vi "Example Zoom.vi"() -> ()   [LabVIEW 2020, in "LcPictureBox.lvclass"]
uses:
  LcPictureBox.lvclass
  System.Windows.Forms
  <vilib>/Utility/miscctls.llb/LVPoint32TypeDef.ctl
  Pen.ctl
  SmoothingMode.ctl
panel:
  in  "PictureBox":refnum<k24>(container)
  out "WheelPosition":cluster{"X":i32, "Y":i32}
  out "MouseDown":cluster{"X":i32, "Y":i32}
  in  "Origin":cluster{"x":sgl, "y":sgl}
  in  "ZoomAtMouse":bool
  out "MousePosition(raw)":cluster{"X":i32, "Y":i32}
  in  "ScaleToFit":bool
  in  "ScaleFactor(1)":dbl=1.0 min=-5.0 max=5.0 step=0.1 format="%#.1f"
  in  "Stop":bool
  out "Updating":u32
  out "Drawing":u32
  out "error out":errorcluster
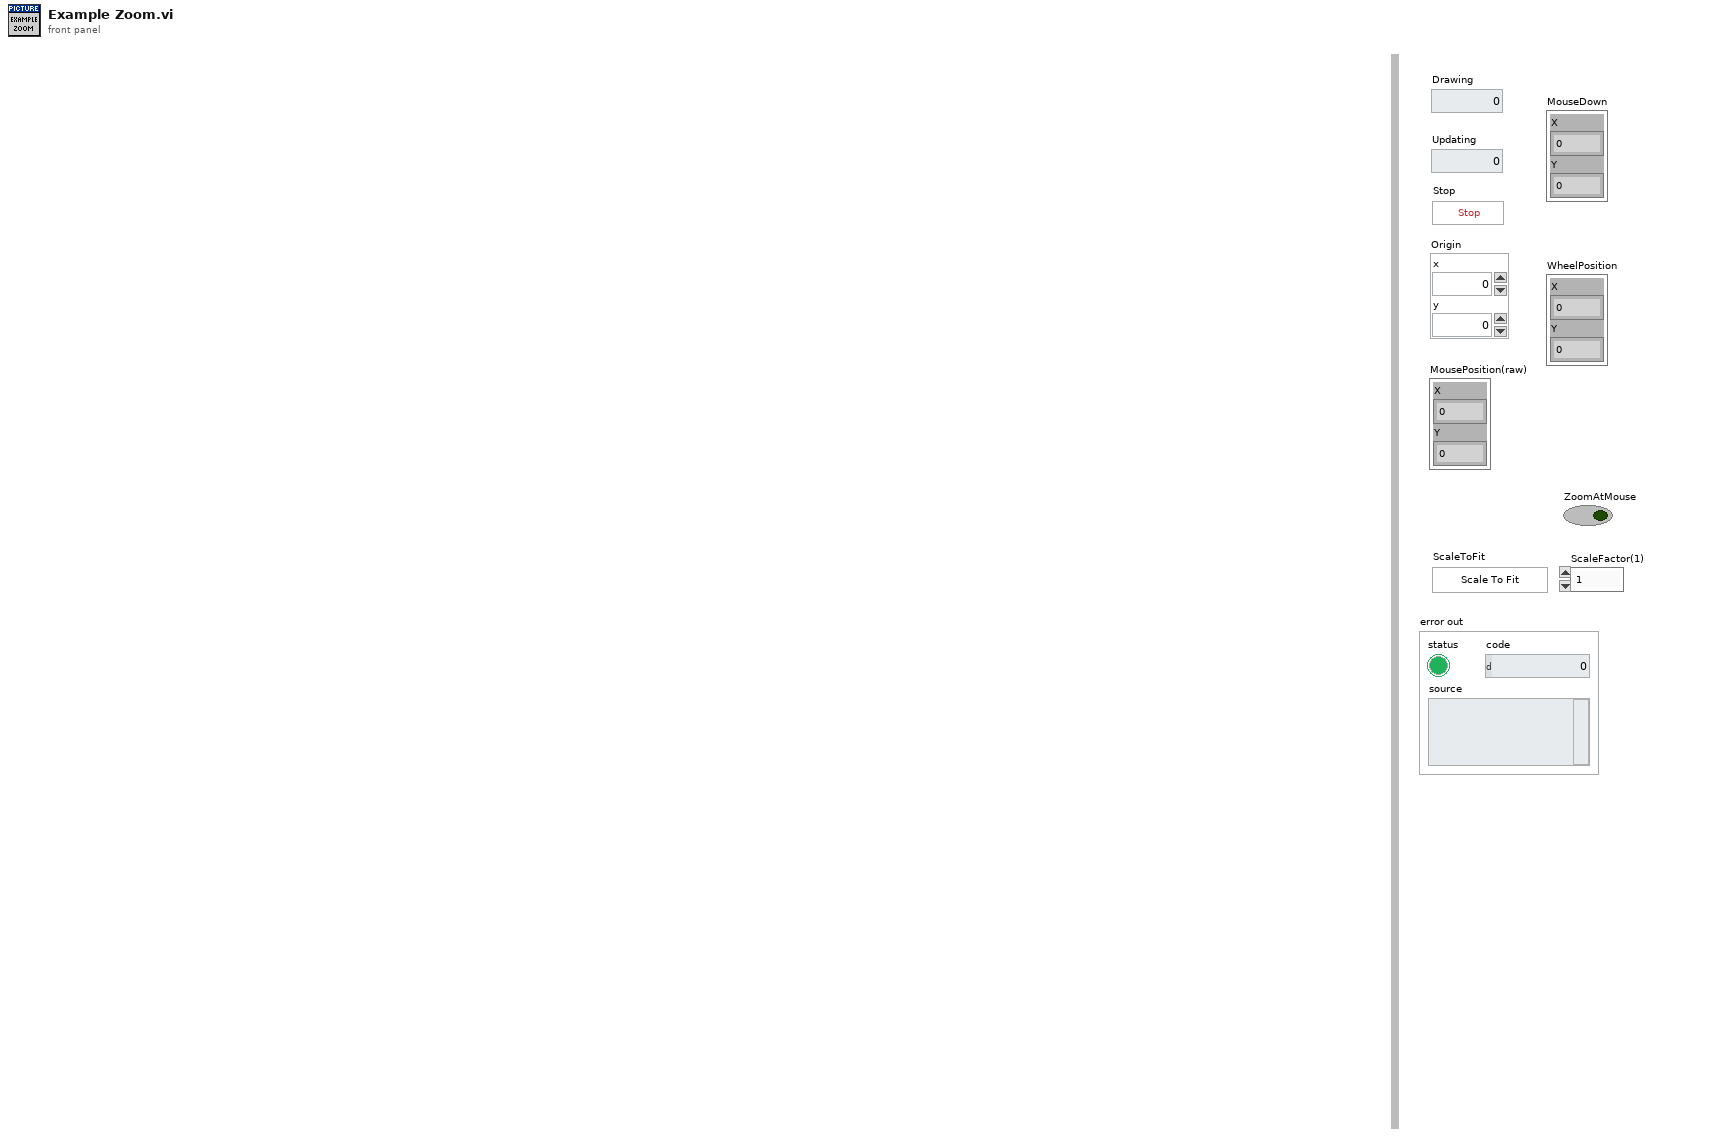
[diagram p1: front panel]
types:
  T1 = typedef "LVPoint32TypeDef.ctl" = cluster{"Horizontal":i32, "Vertical":i32}
  T2 = cluster{"Coords":T1, "MouseDown":bool, "PlatMods":cluster{"Shift":bool, "Ctrl":bool, "Alt":bool, "Cmd":bool, "Opt":bool}}
  T3 = typedef "LcPictureBox.lvclass/Pen.ctl" = cluster{"Width":u16, "Style":enum32{"Solid", "Dash", "Dot", "DashDot", "DashDotDot"}}
  T4 = typedef "LcPictureBox.lvclass/SmoothingMode.ctl" = enum16{"None", "HighSpeed", "HighQuality", "AntiAlias"}
  T5 = cluster{"Shift":bool, "Ctrl":bool, "Alt":bool, "Cmd":bool, "Opt":bool}
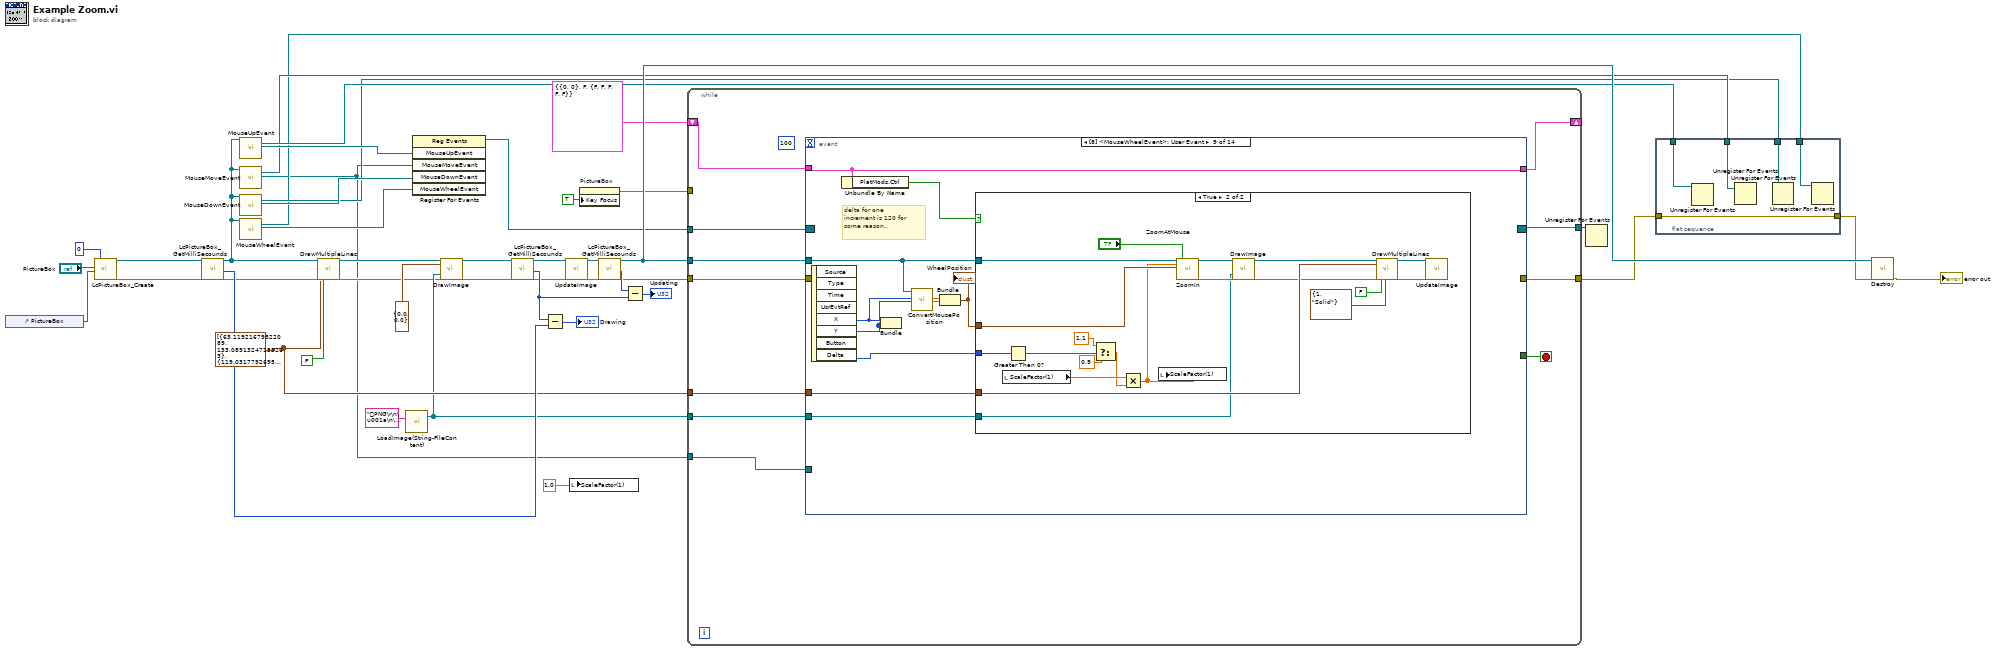
[diagram p0: block diagram]
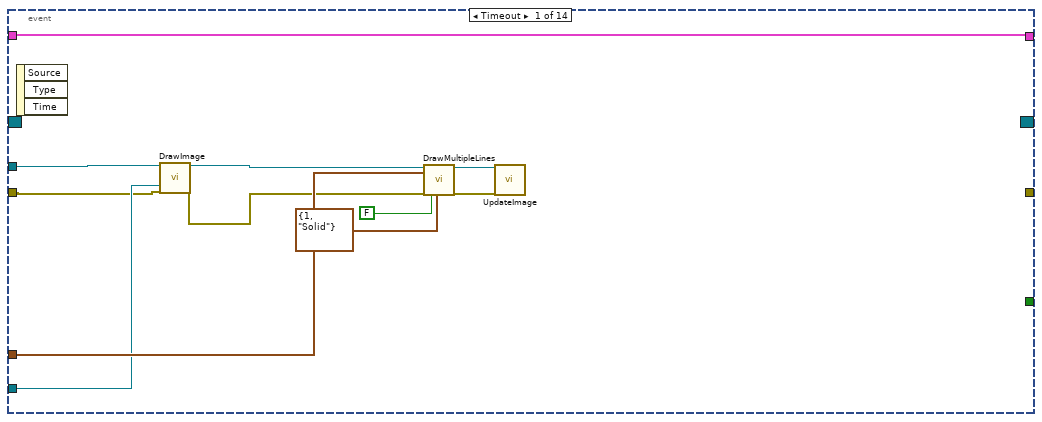
[diagram p2: hidden frame]
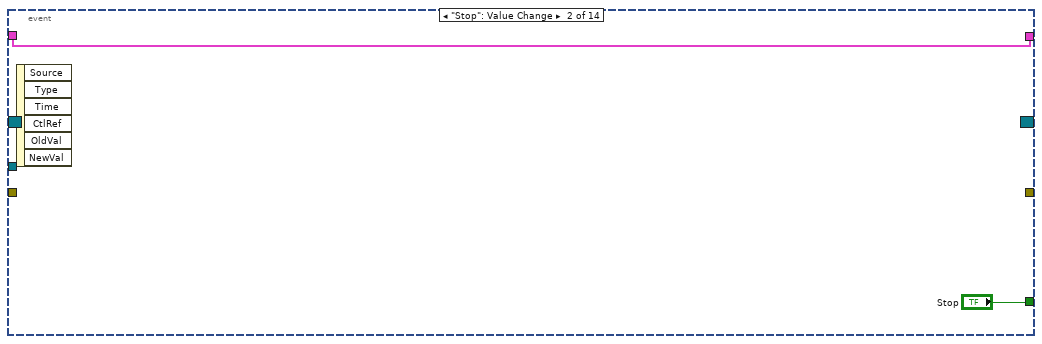
[diagram p3: hidden frame]
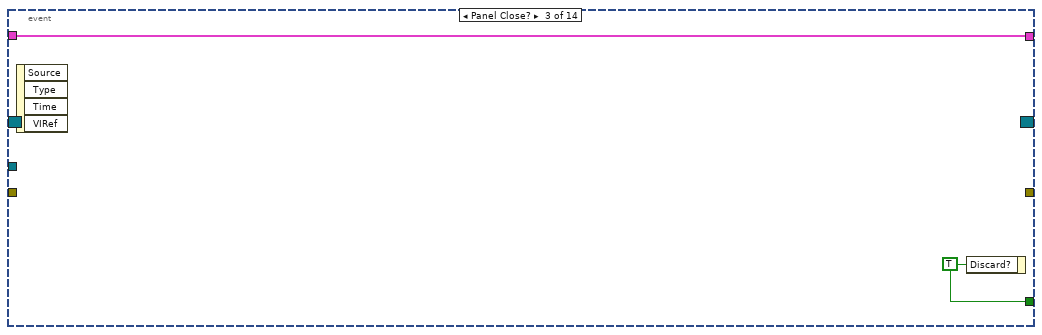
[diagram p4: hidden frame]
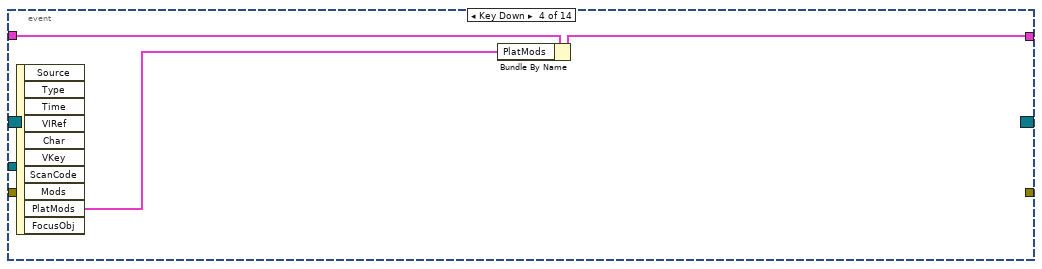
[diagram p5: hidden frame]
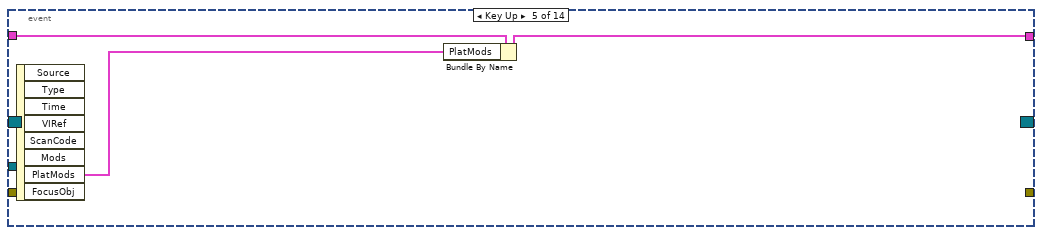
[diagram p6: hidden frame]
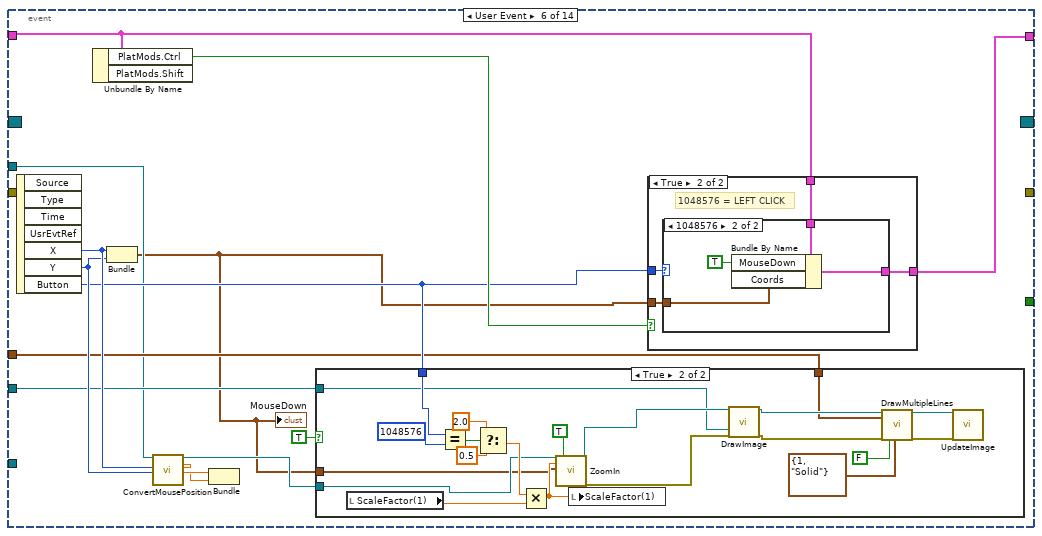
[diagram p7: hidden frame]
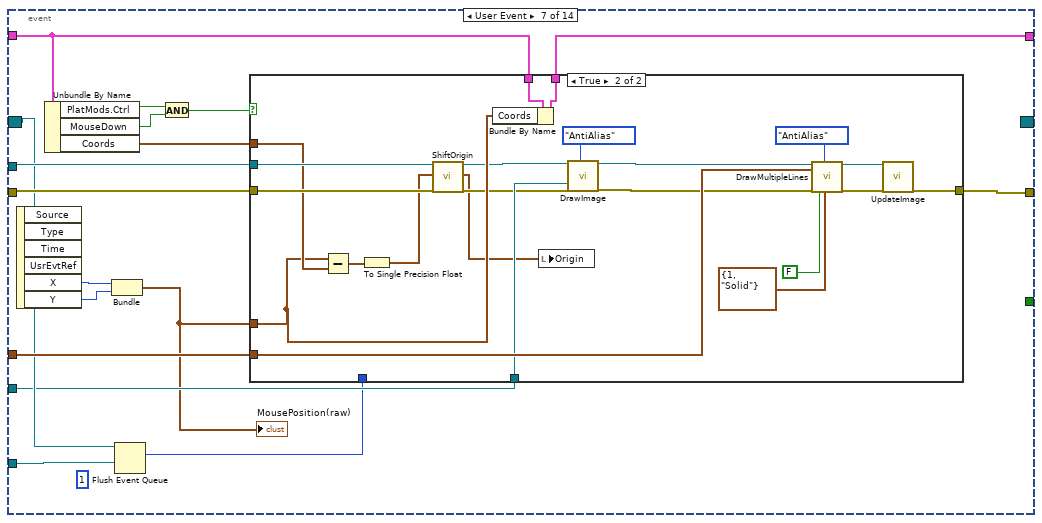
[diagram p11: hidden frame]
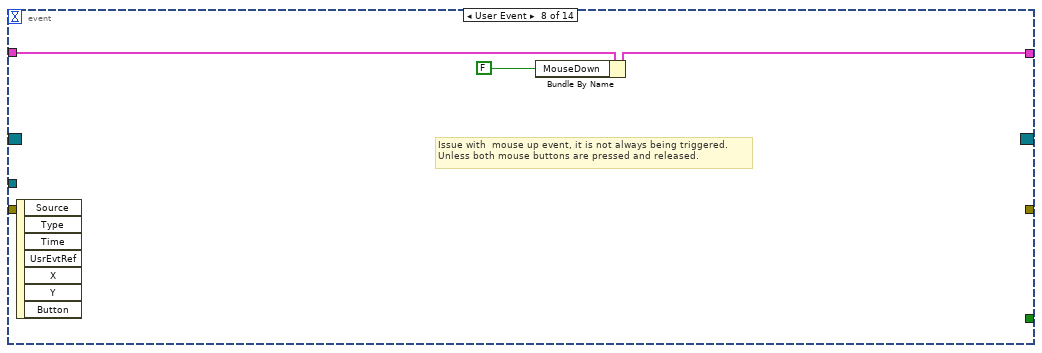
[diagram p13: hidden frame]
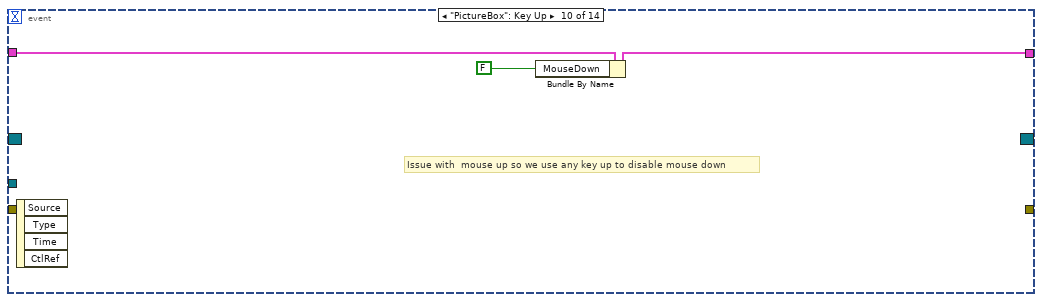
[diagram p15: hidden frame]
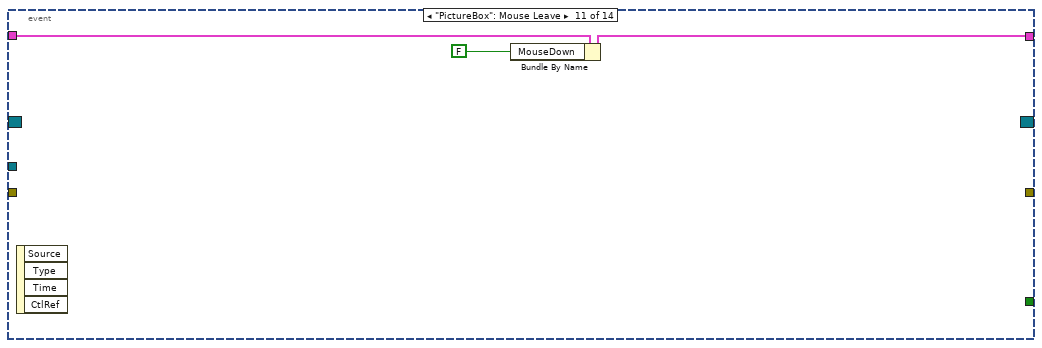
[diagram p16: hidden frame]
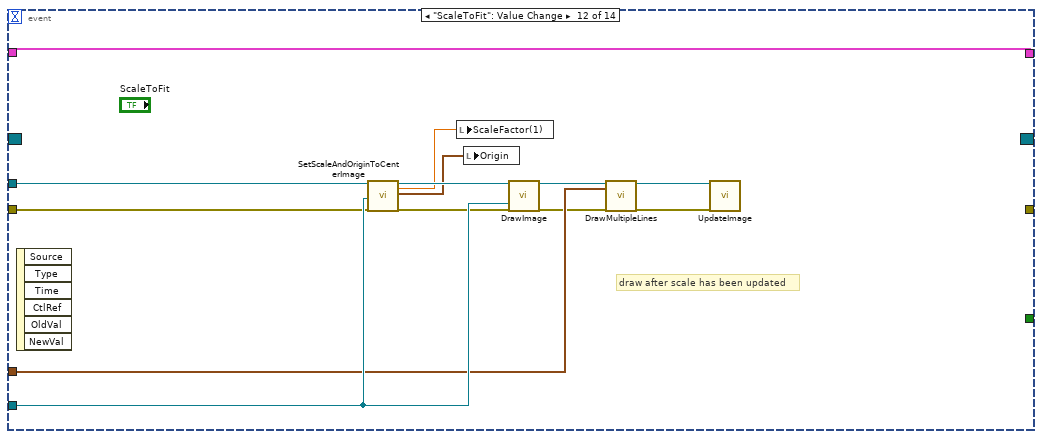
[diagram p17: hidden frame]
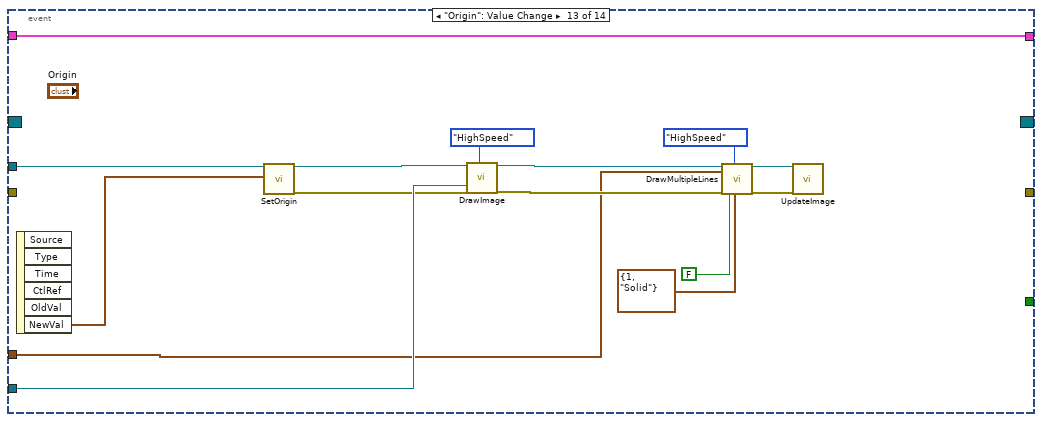
[diagram p18: hidden frame]
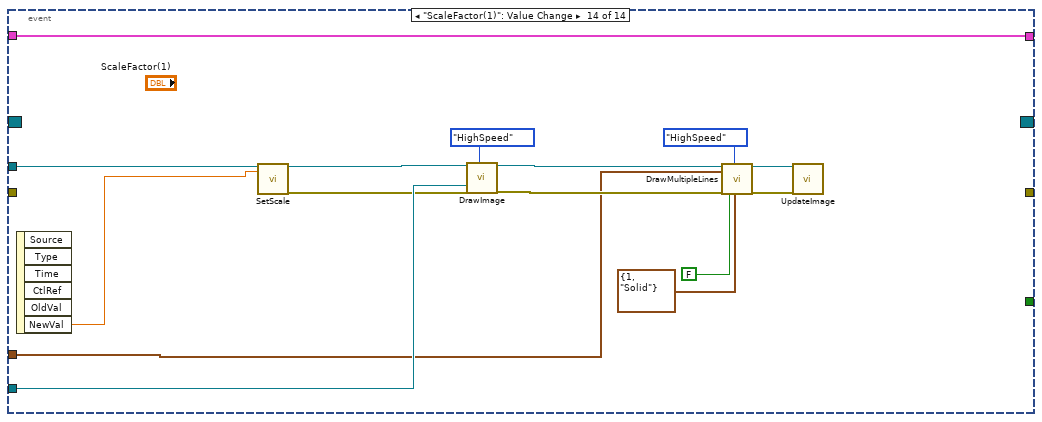
[diagram p19: hidden frame]
diagram:
  w25 = cluster{dbl, dbl}[] [{63.11921679522089, 133.08913247155263}, {119.03177926954152, 161.04541370871294}, {174.94434174386214, 133.08913247155263}, {202.90062298102245, 189.00169494587325}, {174.94434174386214, 244.91425742019388}, {119.03177926954152, 216.95797618303357}, {63.11921679522089, 244.91425742019388}, {35.16293555806058, 189.00169494587325}, {63.11921679522089, 133.08913247155263}]
  n1 = control-ref of="PictureBox"() -> (w39:refnum<vi>)
  n2 = call "LcPictureBox_Create.vi"("PictureBox"="PictureBox", "PictureBoxActiveXReference"=w39, "CacheNumberOfPensAndColors(0)"=0 ("CacheNumberOfPensAndColors(1000)")) -> ("reference out"=w3:refnum<class "LcPictureBox.lvclass">, "Error Out"=w1:errorcluster)  [unwired: 14 in, 1 out]
  n3 = call "LcPictureBox_GetMilliSecounds.vi"("error in (no error)"=w1) -> ("msValue"=w38:u32, "error out"=w31:errorcluster)  [unwired: 17 in]
  n4 = call-dynamic "MouseUpEvent.vi"("reference in"=w3) -> ("Event Callback Refnum"=w15:refnum<k27>, "MouseUpEvent"=w19:refnum<user-event>)  [unwired: 15 in, 2 out]
  n5 = call-dynamic "MouseMoveEvent.vi"("reference in"=w3) -> ("Event Callback Refnum"=w14:refnum<k27>, "MouseMoveEvent"=w4:refnum<user-event>)  [unwired: 15 in, 2 out]
  n6 = call-dynamic "MouseDownEvent.vi"("reference in"=w3) -> ("Event Callback Refnum"=w13:refnum<k27>, "MouseDownEvent"=w18:refnum<user-event>)  [unwired: 15 in, 2 out]
  n7 = call-dynamic "MouseWheelEvent.vi"("reference in"=w3) -> ("Event Callback Refnum"=w9:refnum<k27>, "MouseWheelEvent"=w8:refnum<user-event>)  [unwired: 15 in, 2 out]
  n8 = call-dynamic "DrawMultipleLines.vi"("reference in"=w3, "LineEndPoints"=w25, "Error In"=w31, "Fill(False)"=FALSE ("x > y?")) -> ("reference out"=w28:refnum<class "LcPictureBox.lvclass">, "Error Out"=w6:errorcluster)  [unwired: 14 in]
  n9 = call "LoadImage(String-FileContent).vi"("ImageFileContent"="PNG\r\n\u001a\n\u0000\u0000\u0000\rIHDR\u0000\u0000\u0000ß\u0000\u0000\u0000â\b\u0003\u0000\u0000\u0000ùÃâm\u0000\u0000\u0000PLTEÿÚ\u001cÿÿÿ\u0000\u0000\u0000ÿ×\u0000ÿýôÿÙ\u0000ÿá\u001dÿÝ\u001cÿß\u001d¡\u0012n\u000eUI\tÉ¬\u0016îÌ\u001aÿã\u001dÿÚ\u0015:1\u0006¼ \u0015ÿùãÿäoÿìÿï²ÿý÷ÿÞBÿûîÿ÷Ûÿð¸ÿôÉÿöÔÿåzÿêÿéÿæÿá_ÿßKÿí©ÿòÀÿÞGÿàTÿÜ2ÿêÿäsÿùáöÓ\u001b\u0011we\rÿÝ8ÿâfl\\\f'!\u0004J?\btÙ\u0000\u0000\u0006\u0001IDATxíÝSÓL\u0010\u0007ð«á@}(\u0014ÆÒP\u0014\u0015Ô÷ÿâ\\[´K²¹ìÞþ\u0018¿ÿ1Óéä3´ý6Éºí¸Ý\u001föªéòqu}~~}u²¼<æ:&Ììø¦w÷¾ÜÆûâä#ßqaå¯ªi®²øª^øä\u0015.\u0012_,÷X\u000fot¶¾(ÏpësÏ_»ÂÅ\u0019ï1ÉÆ÷Å·òÐ_2\u001fez6¾NÞZøù8S³öMû|A8å>Ô¤¬}\u001dï¾]ágîMHðUý¿¾°Ô'\f¾9Ð\u0017§Ü\u0007<0Á\u0007æÕÿÒx7ã>äA©}\u0017\u0003|AxwÃ}Ð\u0003â@zµï\nòéùLøPq\u001f80nÐÛoGx®Cè&{mÿZ÷\bëOÜ\u0007\u000fH²/\bW\u0017Üß\u0011¾ ¼ºç\u0006ôd/\b\u001fe×4#}Ax\"Y8Ú'¼¦Að\u0011.Uâ\u0013\\Ó ùÄÖ4h¾0\u0000\u000b\u0014\"úD\u0016Q¨>5\r²O\u0010Ý'¬\"ðªiH|µÐ\t\u0011\u0012ùÄ\u0014QT>)5\rOFMCéPÓÐúðµ¦¡öq\u0017Qô>Þ\"*...") -> ("ImageOut"=w7:refnum<k24>)  [unwired: 16 in, 2 out]
  n10 = register-events(w19, w4, w18, w8) -> (reference out=w17:refnum<event-registration>)  [unwired: 2 in, 1 out]
  n11 = call-dynamic "DrawImage.vi"("reference in"=w28, "UpperLeftCorner(0,0)"=cluster{"x":sgl, "y":sgl} {"x"=0.0, "y"=0.0} ("UpperLeftCorner"), "Image"=w7, "Error In"=w6) -> ("reference out"=w27:refnum<class "LcPictureBox.lvclass">, "Error Out"=w5:errorcluster)  [unwired: 14 in]
  n12 = call "LcPictureBox_GetMilliSecounds.vi"("error in (no error)"=w5) -> ("msValue"=w37:u32, "error out"=w33:errorcluster)  [unwired: 17 in]
  n13 = Subtract(x=w37, y=w38) -> (x-y=→"Drawing":u32)
  n14 = call-dynamic "UpdateImage.vi"("reference in"=w27, "Error In"=w33) -> ("reference out"=w24:refnum<class "LcPictureBox.lvclass">, "Error Out"=w34:errorcluster)  [unwired: 14 in, 2 out]
  n15 = local write "ScaleFactor(1)"(1.0 ("ScaleFactor(1)")) -> ()
  n16 = property on="PictureBox" class="AXCont"("Key Focus"=TRUE) -> (error out=w20:errorcluster)  [unwired: 2 in, 1 out]
  n17 = call "LcPictureBox_GetMilliSecounds.vi"("error in (no error)"=w34) -> ("msValue"=w36:u32, "error out"=w23:errorcluster)  [unwired: 17 in]
  n18 = Subtract(x=w36, y=w37) -> (x-y=→"Updating":u32)
  n19 = while {
    tunnel: w24 -> [w51]
    tunnel: w25 -> [w50]
    tunnel: w7 -> [w49]
    tunnel: w23 -> [w48]
    tunnel: [w47] -> w11
    shift-right: [w46] -> _
    shift-left: T2 {"Coords"={"Horizontal"=0, "Vertical"=0}, "MouseDown"=FALSE, "PlatMods"={"Shift"=FALSE, "Ctrl"=FALSE, "Alt"=FALSE, "Cmd"=FALSE, "Opt"=FALSE}} -> [w44]
    tunnel: w20 -> [_]
    tunnel: w17 -> [w43]
    tunnel: [w45] -> w16
    tunnel: w4 -> [w42]
    stop <- w52 stop-if-true
    (unwired) 100
    n20 = event shown="[8] <MouseWheelEvent>: User Event" {
      selector: w43 -> [_ _ _ _ _ _ w122 _ _ _ _ _ _ _]
      dyn-events: [_ _ _ _ _ _ _ _ _ _ _ _ _ _] -> w45
      timeout: _ -> [_ _ _ _ _ _ _ _ _ _ _ _ _ _]
      tunnel: [_ "Stop" w66 _ _ _ _ _ _ _ _ _ _ _] -> w52
      tunnel: w51 -> [w57 _ _ _ _ w79 w135 _ w167 _ _ w206 w215 w231]
      tunnel: w50 -> [w61 _ _ _ _ w80 w128 _ w173 _ _ w203 w217 w232]
      tunnel: w49 -> [w56 _ _ _ _ w81 w121 _ w170 _ _ w209 w218 w233]
      tunnel: w48 -> [w55 _ _ _ _ _ w134 _ _ _ _ w207 _ _]
      tunnel: [_ _ _ _ _ _ w133 _ _ _ _ _ _ _] -> w47
      tunnel: [w58 w64 w67 w69 w72 w87 w130 w161 w172 w195 w198 w212 w227 w242] -> w46
      tunnel: w44 -> [w58 w64 w67 w70 w73 w86 w127 w162 w172 w196 w199 w212 w227 w242]
      tunnel: w42 -> [_ _ _ _ _ _ w123 _ _ _ _ _ _ _]
      event Timeout {
        n21 = event-data() -> ()  [unwired: 1 in, 3 out]
        n22 = call-dynamic "DrawImage.vi"("reference in"=w57, "Image"=w56, "Error In"=w55) -> ("reference out"=w53:refnum<class "LcPictureBox.lvclass">, "Error Out"=w54:errorcluster)  [unwired: 15 in]
        n23 = call-dynamic "DrawMultipleLines.vi"("reference in"=w53, "LineEndPoints"=w61, "Error In"=w54, "Fill(False)"=FALSE ("x > y?"), "Pen(Width=1, Solid)"=T3 {"Width"=1, "Style"=enum."Solid"}) -> ("reference out"=w60:refnum<class "LcPictureBox.lvclass">, "Error Out"=w59:errorcluster)  [unwired: 13 in]
        n24 = call-dynamic "UpdateImage.vi"("reference in"=w60, "Error In"=w59) -> ()  [unwired: 14 in, 4 out]
      }
      event "Stop": Value Change {
        n25 = event-data() -> ()  [unwired: 1 in, 6 out]
      }
      event Panel Close? {
        w66 = TRUE ("Discard?")
        n26 = event-data() -> ()  [unwired: 1 in, 4 out]
        n27 = event-data("Discard?"=w66) -> ()  [unwired: 1 in, 1 out]
      }
      event Key Down {
        n28 = event-data() -> ("PlatMods"=w68:T5)  [unwired: 1 in, 9 out]
        n29 = Bundle By Name(cluster=w70, "PlatMods"=w68) -> (w69:T2)
      }
      event Key Up {
        n30 = event-data() -> ("PlatMods"=w71:T5)  [unwired: 1 in, 7 out]
        n31 = Bundle By Name(cluster=w73, "PlatMods"=w71) -> (w72:T2)
      }
      event User Event {
        n32 = event-data() -> ("X"=w84:i32, "Y"=w83:i32, "Button"=w82:i32)  [unwired: 1 in, 4 out]
        n33 = Unbundle By Name(w86) -> ("PlatMods.Ctrl"=w85:bool)  [unwired: 1 out]
        n34 = Bundle("X"=w84, "Y"=w83) -> (w74:cluster{"X":i32, "Y":i32})  [unwired: 1 in]
        "MouseDown" <- w74
        n35 = call-dynamic "ConvertMousePosition.vi"("reference in"=w79, "X"=w84, "Y"=w83) -> ("reference out"=w78:refnum<class "LcPictureBox.lvclass">, "X-Out"=w77:sgl, "Y-Out"=w76:sgl)  [unwired: 13 in, 1 out]
        n36 = Bundle("X-Out"=w77, "Y-Out"=w76) -> ()  [unwired: 1 in, 1 out]
        n37 = case shown="True" TRUE {
          tunnel: w82 -> [_ w104]
          tunnel: w81 -> [_ w91]
          tunnel: w80 -> [_ w90]
          tunnel: w78 -> [_ w89]
          tunnel: w74 -> [_ w88]
          frame False {
          }
          frame True {
            n38 = local read "ScaleFactor(1)"() -> (w100:dbl)
            n39 = Equal?(x=w104, y=1048576) -> (x = y?=w107:bool)
            n40 = Select(t=2.0, s=w107, f=0.5) -> (s? t:f=w102:dbl)
            n41 = Multiply(x=w102, y=w100) -> (x*y=w101:dbl)
            n42 = call-dynamic "ZoomIn.vi"("reference in"=w89, "NewScaleValue"=w101, "MousePosition(scaled)"=w88, "ZoomAtMouse"=TRUE) -> ("reference out"=w93:refnum<class "LcPictureBox.lvclass">, "Error Out"=w92:errorcluster)  [unwired: 12 in, 2 out]
            n43 = local write "ScaleFactor(1)"(w101) -> ()
            n44 = call-dynamic "DrawImage.vi"("reference in"=w93, "Image"=w91, "Error In"=w92) -> ("reference out"=w94:refnum<class "LcPictureBox.lvclass">, "Error Out"=w95:errorcluster)  [unwired: 15 in]
            n45 = call-dynamic "DrawMultipleLines.vi"("reference in"=w94, "LineEndPoints"=w90, "Error In"=w95, "Fill(False)"=FALSE ("x > y?"), "Pen(Width=1, Solid)"=T3 {"Width"=1, "Style"=enum."Solid"}) -> ("reference out"=w97:refnum<class "LcPictureBox.lvclass">, "Error Out"=w96:errorcluster)  [unwired: 13 in]
            n46 = call-dynamic "UpdateImage.vi"("reference in"=w97, "Error In"=w96) -> ()  [unwired: 14 in, 4 out]
          }
        }
        n47 = case shown="True" w85 {
          tunnel: w86 -> [w109 w113]
          tunnel: [w109 w112] -> w87
          tunnel: w82 -> [_ w111]
          tunnel: w74 -> [_ w110]
          frame False {
          }
          frame True {
            # "1048576 = LEFT CLICK"
            n48 = case shown="1048576" w111 {
              tunnel: w113 -> [w114 w118]
              tunnel: [w114 w117] -> w112
              tunnel: w110 -> [_ w115]
              frame 0, Default {
              }
              frame 1048576 {
                n49 = Bundle By Name(cluster=w118, "MouseDown"=TRUE, "Coords"=w115) -> (w117:T2)
              }
            }
          }
        }
      }
      event User Event {
        (unwired) 1 ("keep most recent")
        n50 = event-data() -> ("X"=w131:i32, "Y"=w132:i32)  [unwired: 1 in, 4 out]
        n51 = Unbundle By Name(w127) -> ("PlatMods.Ctrl"=w126:bool, "MouseDown"=w125:bool, "Coords"=w129:T1)
        n52 = Bundle("X"=w131, "Y"=w132) -> (w119:cluster{"X":i32, "Y":i32})  [unwired: 1 in]
        "MousePosition(raw)" <- w119
        n53 = Flush Event Queue(0:w122, 2:w123) -> (9:w120:u32)  [unwired: 4 in, 2 out]
        n54 = And(x=w126, y=w125) -> (x .and. y?=w124:bool)
        n55 = case shown="True" w124 {
          tunnel: w135 -> [_ w159]
          tunnel: w134 -> [w137 w158]
          tunnel: [w137 w146] -> w133
          tunnel: [w136 w156] -> w130
          tunnel: w127 -> [w136 w157]
          tunnel: w119 -> [_ w154]
          tunnel: w129 -> [_ w155]
          tunnel: w128 -> [_ w147]
          tunnel: w121 -> [_ w143]
          tunnel: w120 -> [_ _]
          frame False {
          }
          frame True {
            n56 = Subtract(x=w154, y=w155) -> (x-y=w153:T1)
            n57 = To Single Precision Float(number=w153) -> (single precision float=w152:cluster{"Horizontal":sgl, "Vertical":sgl})
            n58 = call-dynamic "ShiftOrigin.vi"("reference in"=w159, "Delta(raw)"=w152, "Error In"=w158) -> ("reference out"=w144:refnum<class "LcPictureBox.lvclass">, "Origin"=w138:cluster{"x":sgl, "y":sgl}, "Error Out"=w142:errorcluster)  [unwired: 14 in]
            n59 = Bundle By Name(cluster=w157, "Coords"=w154) -> (w156:T2)
            n60 = local write "Origin"(w138) -> ()
            n61 = call-dynamic "DrawImage.vi"("reference in"=w144, "Image"=w143, "Error In"=w142, "SmoothingMode(AntiAlias)"=SmoothingMode."AntiAlias" ("SmoothingMode")) -> ("reference out"=w141:refnum<class "LcPictureBox.lvclass">, "Error Out"=w140:errorcluster)  [unwired: 14 in]
            n62 = call-dynamic "DrawMultipleLines.vi"("reference in"=w141, "LineEndPoints"=w147, "Error In"=w140, "Fill(False)"=FALSE ("x > y?"), "SmoothingMode(AntiAlias)"=SmoothingMode."AntiAlias", "Pen(Width=1, Solid)"=T3 {"Width"=1, "Style"=enum."Solid"}) -> ("reference out"=w149:refnum<class "LcPictureBox.lvclass">, "Error Out"=w148:errorcluster)  [unwired: 12 in]
            n63 = call-dynamic "UpdateImage.vi"("reference in"=w149, "Error In"=w148) -> ("Error Out"=w146:errorcluster)  [unwired: 14 in, 3 out]
          }
        }
      }
      event User Event {
        # "Issue with  mouse up event, it is not always being triggered.\nUnless both mouse buttons are pressed and released."
        n64 = event-data() -> ()  [unwired: 1 in, 7 out]
        n65 = Bundle By Name(cluster=w162, "MouseDown"=FALSE) -> (w161:T2)
      }
      event User Event {
        # "delta for one increment is 120 for some reason.."
        n66 = event-data() -> ("X"=w169:i32, "Y"=w168:i32, "Delta"=w163:i32)  [unwired: 1 in, 5 out]
        n67 = Unbundle By Name(w172) -> ("PlatMods.Ctrl"=w171:bool)
        n68 = Bundle("X"=w169, "Y"=w168) -> ()  [unwired: 1 in, 1 out]
        n69 = call-dynamic "ConvertMousePosition.vi"("reference in"=w167, "X"=w169, "Y"=w168) -> ("X-Out"=w166:sgl, "Y-Out"=w164:sgl)  [unwired: 13 in, 2 out]
        n70 = Bundle("X-Out"=w166, "Y-Out"=w164) -> (w165:cluster{"X-Out":sgl, "Y-Out":sgl})  [unwired: 1 in]
        "WheelPosition" <- w165
        n71 = case shown="True" w171 {
          tunnel: w167 -> [_ w188]
          tunnel: w173 -> [_ w189]
          tunnel: w165 -> [_ w187]
          tunnel: w170 -> [_ w184]
          tunnel: w163 -> [_ w178]
          frame False {
          }
          frame True {
            n72 = local read "ScaleFactor(1)"() -> (w176:dbl)
            n73 = Greater Than 0?(x=w178) -> (x > 0?=w177:bool)
            n74 = Select(t=1.1, s=w177, f=0.9) -> (s? t:f=w175:dbl)
            n75 = Multiply(x=w176, y=w175) -> (x*y=w174:dbl)
            n76 = local write "ScaleFactor(1)"(w174) -> ()
            n77 = call-dynamic "ZoomIn.vi"("reference in"=w188, "NewScaleValue"=w174, "MousePosition(scaled)"=w187, "ZoomAtMouse"="ZoomAtMouse") -> ("reference out"=w186:refnum<class "LcPictureBox.lvclass">, "Error Out"=w185:errorcluster)  [unwired: 12 in, 2 out]
            n78 = call-dynamic "DrawImage.vi"("reference in"=w186, "Image"=w184, "Error In"=w185) -> ("reference out"=w182:refnum<class "LcPictureBox.lvclass">, "Error Out"=w183:errorcluster)  [unwired: 15 in]
            n79 = call-dynamic "DrawMultipleLines.vi"("reference in"=w182, "LineEndPoints"=w189, "Error In"=w183, "Fill(False)"=FALSE ("x > y?"), "Pen(Width=1, Solid)"=T3 {"Width"=1, "Style"=enum."Solid"}) -> ("reference out"=w191:refnum<class "LcPictureBox.lvclass">, "Error Out"=w190:errorcluster)  [unwired: 13 in]
            n80 = call-dynamic "UpdateImage.vi"("reference in"=w191, "Error In"=w190) -> ()  [unwired: 14 in, 4 out]
          }
        }
      }
      event "PictureBox": Key Up {
        # "Issue with  mouse up so we use any key up to disable mouse down"
        n81 = event-data() -> ()  [unwired: 1 in, 4 out]
        n82 = Bundle By Name(cluster=w196, "MouseDown"=FALSE) -> (w195:T2)
      }
      event "PictureBox": Mouse Leave {
        n83 = event-data() -> ()  [unwired: 1 in, 4 out]
        n84 = Bundle By Name(cluster=w199, "MouseDown"=FALSE) -> (w198:T2)
      }
      event "ScaleToFit": Value Change {
        # "draw after scale has been updated"
        n85 = event-data() -> ()  [unwired: 1 in, 6 out]
        n86 = call-dynamic "SetScaleAndOriginToCenterImage.vi"("reference in"=w206, "Image"=w209, "Error In"=w207) -> ("reference out"=w211:refnum<class "LcPictureBox.lvclass">, "ScaleFactorUsed"=w210:sgl, "OriginUsed"=w200:cluster{"x":sgl, "y":sgl}, "Error Out"=w208:errorcluster)  [unwired: 13 in]
        n87 = local write "ScaleFactor(1)"(w210) -> ()
        n88 = local write "Origin"(w200) -> ()
        n89 = call-dynamic "DrawImage.vi"("reference in"=w211, "Image"=w209, "Error In"=w208) -> ("reference out"=w205:refnum<class "LcPictureBox.lvclass">, "Error Out"=w202:errorcluster)  [unwired: 15 in]
        n90 = call-dynamic "DrawMultipleLines.vi"("reference in"=w205, "LineEndPoints"=w203, "Error In"=w202) -> ("reference out"=w204:refnum<class "LcPictureBox.lvclass">, "Error Out"=w201:errorcluster)  [unwired: 15 in]
        n91 = call-dynamic "UpdateImage.vi"("reference in"=w204, "Error In"=w201) -> ()  [unwired: 14 in, 4 out]
      }
      event "Origin": Value Change {
        n92 = event-data() -> ("NewVal"=w216:cluster{"x":sgl, "y":sgl})  [unwired: 1 in, 5 out]
        n93 = call-dynamic "SetOrigin.vi"("reference in"=w215, "Origin"=w216) -> ("reference out"=w214:refnum<class "LcPictureBox.lvclass">, "Error Out"=w213:errorcluster)  [unwired: 16 in]
        n94 = call-dynamic "DrawImage.vi"("reference in"=w214, "Image"=w218, "Error In"=w213, "SmoothingMode(AntiAlias)"=SmoothingMode."HighSpeed" ("SmoothingMode")) -> ("reference out"=w221:refnum<class "LcPictureBox.lvclass">, "Error Out"=w220:errorcluster)  [unwired: 14 in]
        n95 = call-dynamic "DrawMultipleLines.vi"("reference in"=w221, "LineEndPoints"=w217, "Error In"=w220, "Fill(False)"=FALSE ("x > y?"), "SmoothingMode(AntiAlias)"=SmoothingMode."HighSpeed", "Pen(Width=1, Solid)"=T3 {"Width"=1, "Style"=enum."Solid"}) -> ("reference out"=w224:refnum<class "LcPictureBox.lvclass">, "Error Out"=w223:errorcluster)  [unwired: 12 in]
        n96 = call-dynamic "UpdateImage.vi"("reference in"=w224, "Error In"=w223) -> ()  [unwired: 14 in, 4 out]
      }
      event "ScaleFactor(1)": Value Change {
        n97 = event-data() -> ("NewVal"=w229:dbl)  [unwired: 1 in, 5 out]
        n98 = call-dynamic "SetScale.vi"("reference in"=w231, "ScaleFactor"=w229) -> ("reference out"=w230:refnum<class "LcPictureBox.lvclass">, "Error Out"=w228:errorcluster)  [unwired: 16 in]
        n99 = call-dynamic "DrawImage.vi"("reference in"=w230, "Image"=w233, "Error In"=w228, "SmoothingMode(AntiAlias)"=SmoothingMode."HighSpeed" ("SmoothingMode")) -> ("reference out"=w236:refnum<class "LcPictureBox.lvclass">, "Error Out"=w235:errorcluster)  [unwired: 14 in]
        n100 = call-dynamic "DrawMultipleLines.vi"("reference in"=w236, "LineEndPoints"=w232, "Error In"=w235, "Fill(False)"=FALSE ("x > y?"), "SmoothingMode(AntiAlias)"=SmoothingMode."HighSpeed", "Pen(Width=1, Solid)"=T3 {"Width"=1, "Style"=enum."Solid"}) -> ("reference out"=w239:refnum<class "LcPictureBox.lvclass">, "Error Out"=w238:errorcluster)  [unwired: 12 in]
        n101 = call-dynamic "UpdateImage.vi"("reference in"=w239, "Error In"=w238) -> ()  [unwired: 14 in, 4 out]
      }
    }
  }
  n102 = Unregister For Events(event registration refnum=w16) -> ()  [unwired: 1 in, 1 out]
  n103 = flat-sequence {
    tunnel: w15 -> [w247]
    tunnel: w14 -> [w246]
    tunnel: w13 -> [w245]
    tunnel: [w244] -> w10
    tunnel: w11 -> [w244]
    tunnel: w9 -> [w243]
    frame #0 {
      n104 = Unregister For Events(event registration refnum=w247) -> ()  [unwired: 1 in, 1 out]
      n105 = Unregister For Events(event registration refnum=w246) -> ()  [unwired: 1 in, 1 out]
      n106 = Unregister For Events(event registration refnum=w245) -> ()  [unwired: 1 in, 1 out]
      n107 = Unregister For Events(event registration refnum=w243) -> ()  [unwired: 1 in, 1 out]
    }
  }
  n108 = call-dynamic "Destroy.vi"("reference in"=w24, "Error In"=w10) -> ("Error Out"=→"error out":errorcluster)  [unwired: 16 in, 1 out]
